vi "NI_9219_Config.vi"(8 "error in":errorcluster, 11 "task in":refnum<k21>) -> (0 "error out":errorcluster, 3 "task out":refnum<k21>)   [LabVIEW 2022 SP3]
uses:
  <vilib>/DAQmx/create/channels.llb/DAQmx Create Channel (AI-Voltage-Basic).vi
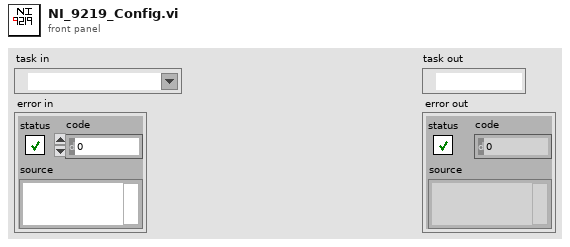
[diagram p1: front panel]
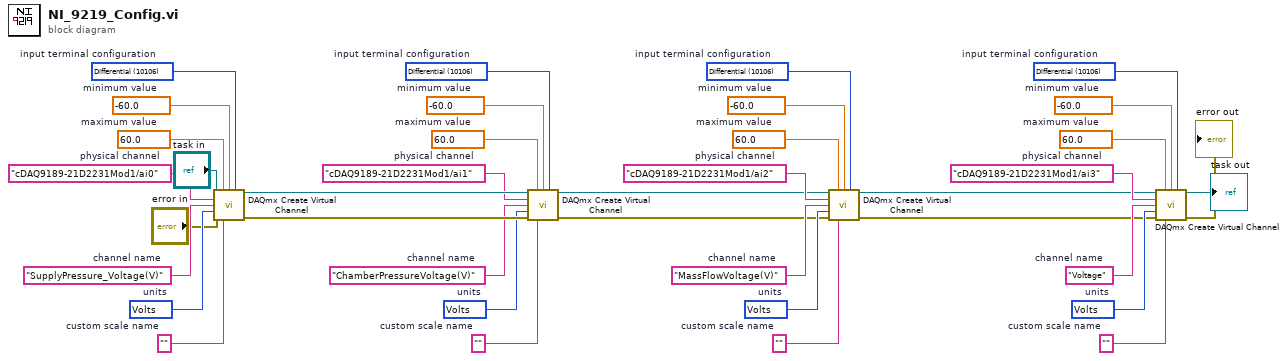
[diagram p0: block diagram]
diagram:
  w5 = 10106 items=["default"=-1, "RSE"=10083, "NRSE"=10078, "Differential"=10106, "Pseudodifferential"=12529]  # input terminal configuration
  w6 = 10348 items=["Volts"=10348, "From Custom Scale"=10065]  # units
  w7 = "MassFlowVoltage(V)"  # channel name
  w8 = ""  # custom scale name
  w9 = -60.0  # minimum value
  w10 = 60.0  # maximum value
  w11 = "cDAQ9189-21D2231Mod1/ai2"  # physical channel
  w16 = 10106 items=["default"=-1, "RSE"=10083, "NRSE"=10078, "Differential"=10106, "Pseudodifferential"=12529]  # input terminal configuration
  w17 = 10348 items=["Volts"=10348, "From Custom Scale"=10065]  # units
  w18 = "Voltage"  # channel name
  w19 = ""  # custom scale name
  w20 = -60.0  # minimum value
  w21 = 60.0  # maximum value
  w22 = "cDAQ9189-21D2231Mod1/ai3"  # physical channel
  w23 = 10106 items=["default"=-1, "RSE"=10083, "NRSE"=10078, "Differential"=10106, "Pseudodifferential"=12529]  # input terminal configuration
  w24 = 10348 items=["Volts"=10348, "From Custom Scale"=10065]  # units
  w25 = "ChamberPressureVoltage(V)"  # channel name
  w26 = ""  # custom scale name
  w27 = -60.0  # minimum value
  w28 = 60.0  # maximum value
  w29 = "cDAQ9189-21D2231Mod1/ai1"  # physical channel
  w31 = 10106 items=["default"=-1, "RSE"=10083, "NRSE"=10078, "Differential"=10106, "Pseudodifferential"=12529]  # input terminal configuration
  w32 = 10348 items=["Volts"=10348, "From Custom Scale"=10065]  # units
  w33 = "SupplyPressure_Voltage(V)"  # channel name
  w35 = ""  # custom scale name
  w36 = -60.0  # minimum value
  w37 = 60.0  # maximum value
  w38 = "cDAQ9189-21D2231Mod1/ai0"  # physical channel
  n1 = call-poly <vilib>:"DAQmx Create Virtual Channel.vi"("task in"="task in", "maximum value"=w37, "minimum value"=w36, "input terminal configuration"=w31, "physical channels"=w38, "name to assign"=w33, "units"=w32, "error in"="error in", "custom scale name"=w35) -> ("task out"=w30:refnum<k21>, "error out"=w34:errorcluster)  [unwired: 5 in]
  n2 = call-poly <vilib>:"DAQmx Create Virtual Channel.vi"("task in"=w30, "maximum value"=w28, "minimum value"=w27, "input terminal configuration"=w23, "physical channels"=w29, "name to assign"=w25, "units"=w24, "error in"=w34, "custom scale name"=w26) -> ("task out"=w4:refnum<k21>, "error out"=w3:errorcluster)  [unwired: 5 in]
  n3 = call-poly <vilib>:"DAQmx Create Virtual Channel.vi"("task in"=w4, "maximum value"=w10, "minimum value"=w9, "input terminal configuration"=w5, "physical channels"=w11, "name to assign"=w7, "units"=w6, "error in"=w3, "custom scale name"=w8) -> ("task out"=w1:refnum<k21>, "error out"=w2:errorcluster)  [unwired: 5 in]
  n4 = call-poly <vilib>:"DAQmx Create Virtual Channel.vi"("task in"=w1, "maximum value"=w21, "minimum value"=w20, "input terminal configuration"=w16, "physical channels"=w22, "name to assign"=w18, "units"=w17, "error in"=w2, "custom scale name"=w19) -> ("task out"=→"task out":refnum<k21>, "error out"=→"error out":errorcluster)  [unwired: 5 in]
